vi "Laser Ops standalone diagnostics.vi"() -> ()   [LabVIEW 2017]
uses:
  Serial Comms/Visa resource.ctl
  Type Defs/Ls1 Operations.ctl
panel:
  out "Resp Validated (array) ?":bool[](array[boolean])
  out "Tmin":dbl
  out "Tmax":dbl
  out "Laser shutter":bool
  out "Ls Data":string[](array[string])
  out "error out inter":errorcluster
  out "error out":errorcluster
  in  "Program Stop":bool
  out "Pump peak hold":bool
  out "Power [mW]":dbl
  out "Read Wavelength [nm]":dbl
  in  "Laser Shutter":bool
  out "Tuning Status":string
  out "Fault":string
  out "Mode":string
  in  "PreChirper Available ?":bool
  in  "Laser Available ?":bool
  in  "Update":bool
  in  "Wavelength (nm)":u16
  in  "error in (no error)":errorcluster
  in  "PreChrp1 \nVisa resource":T1
  in  "Ls1 Visa \nresource":T1={"VISA resource name"="COM14", "baud rate"=19200}
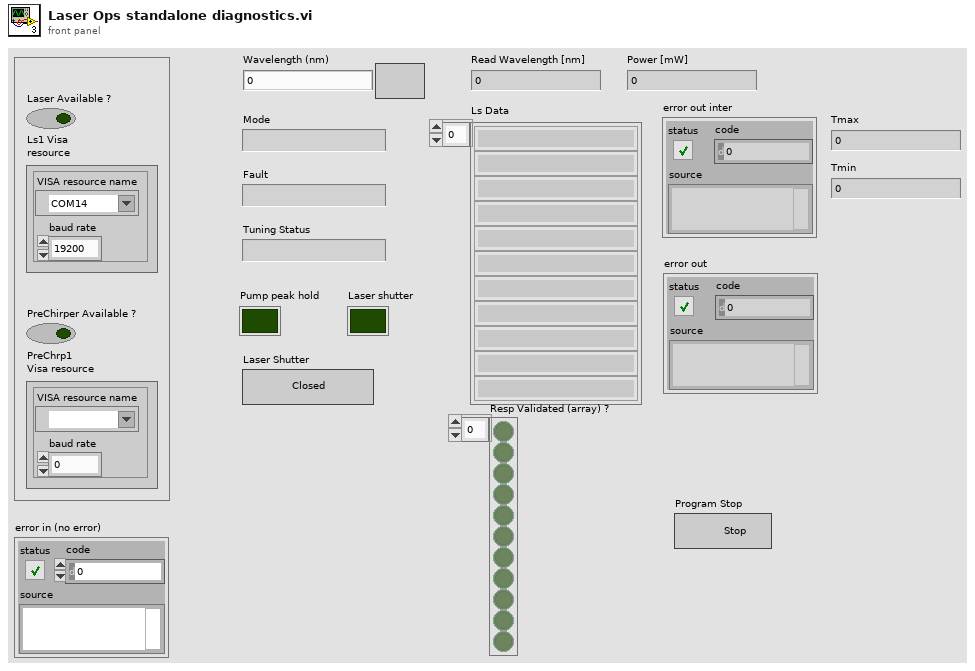
[diagram p1: front panel]
types:
  T1 = typedef "Visa resource.ctl" = cluster{"VISA resource name":refnum<visa-resource-name>, "baud rate":u32}
  T2 = typedef "Ls1 Operations.ctl" = enum16{"Initialise Connections", "Initialise system", "Check Status", "Open/Close Shutter", "Start/Stop Pump Peak Hold", "Set wavelength", "Close"}
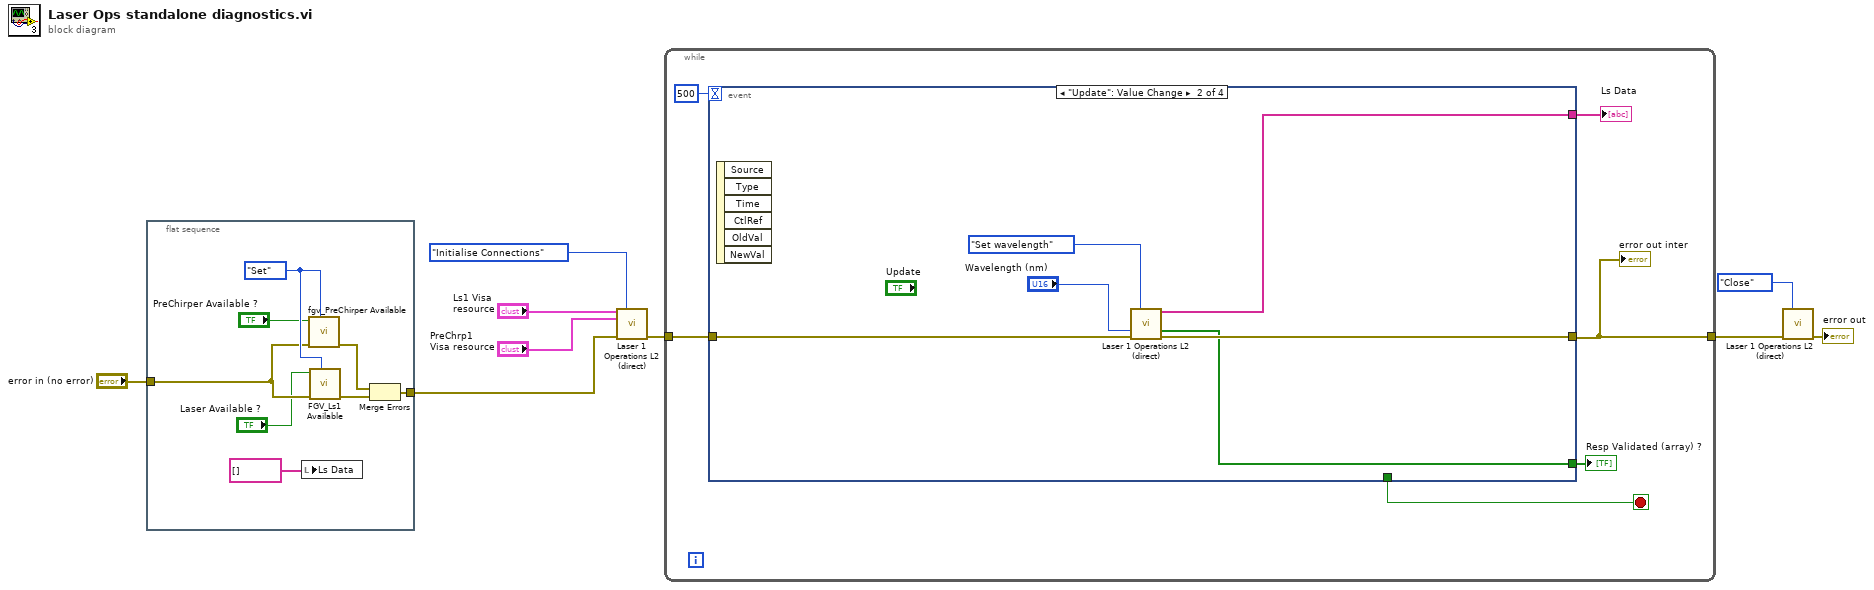
[diagram p0: block diagram]
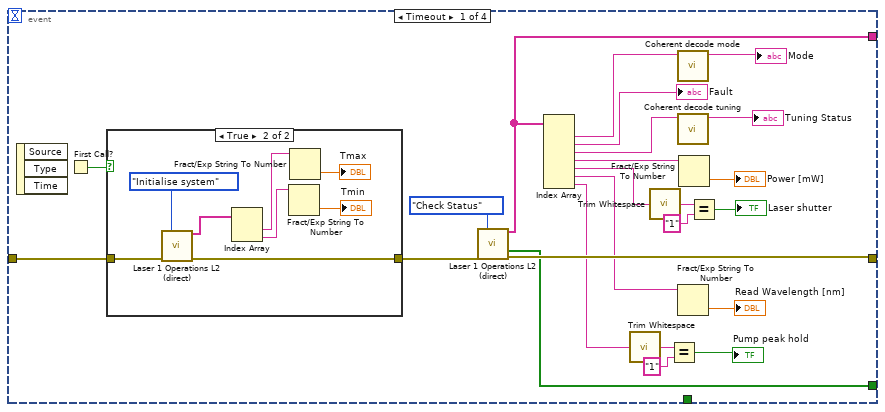
[diagram p2: hidden frame]
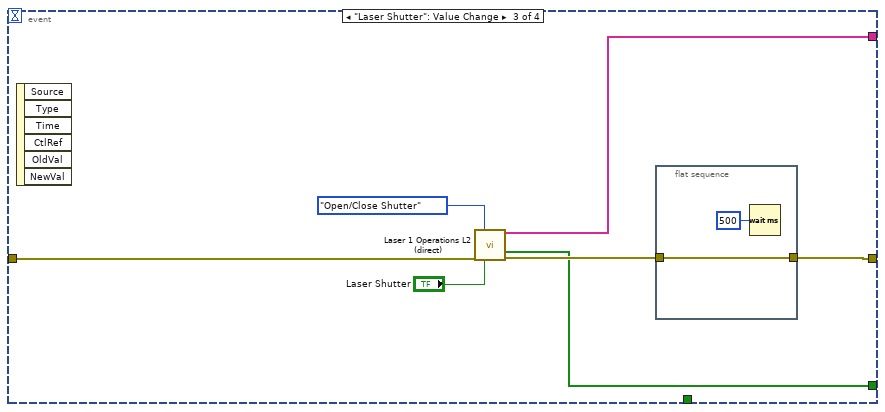
[diagram p4: hidden frame]
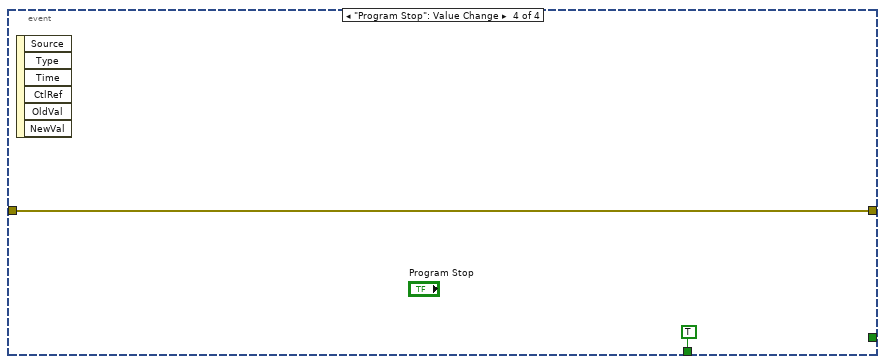
[diagram p5: hidden frame]
diagram:
  n1 = flat-sequence {
    tunnel: "error in (no error)" -> [w15]
    tunnel: [w12] -> w4
    frame #0 {
      w17 = enum16{"Get", "Set"}."Set" ("FGV Actions")
      n2 = local write "Ls Data"(string[] []) -> ()
      n3 = call "fgv_PreChirper Available.vi"("FGV Actions"=w17, "error in (no error)"=w15, "PreChirper Available ? IN"="PreChirper Available ?") -> ("error out"=w13:errorcluster)  [unwired: 7 in, 1 out]
      n4 = call "FGV_Ls1 Available.vi"("FGV Actions"=w17, "error in (no error)"=w15, "Laser Available ? IN"="Laser Available ?") -> ("error out"=w14:errorcluster)  [unwired: 7 in, 1 out]
      n5 = Merge Errors(w13, w14) -> (w12:errorcluster)
    }
  }
  n6 = call "Laser 1 Operations L2 (direct).vi"("Ls1 Visa \nresource"="Ls1 Visa \nresource", "Laser Ops\n actions"=Ls1_Operations."Initialise Connections" ("Laser Ops\n actions"), "PreChrp1 \nVisa resource"="PreChrp1 \nVisa resource", "error in (no error)"=w4) -> ("error out"=w6:errorcluster)  [unwired: 6 in, 5 out]
  n7 = while {
    tunnel: w6 -> [w23]
    tunnel: [w20] -> w2
    stop <- w21 stop-if-true
    n8 = event shown="[1] \"Update\": Value Change" {
      selector: _ -> [_ _ _ _]
      dyn-events: _ -> [_ _ _ _]
      timeout: 500 -> [_ _ _ _]
      tunnel: w23 -> [w46 w62 w68 w72]
      tunnel: [w44 w61 w64 w72] -> w20
      tunnel: [_ _ _ TRUE] -> w21
      tunnel: [w30 w58 w66 _] -> w19
      tunnel: [w24 w57 w63 _] -> w18
      event Timeout {
        n9 = event-data() -> ()  [unwired: 1 in, 3 out]
        n10 = First Call?() -> (First Call?: T/F=w47:bool)
        n11 = case shown="True" w47 {
          tunnel: w46 -> [w48 w56]
          tunnel: [w48 w49] -> w45
          frame False {
          }
          frame True {
            n12 = call "Laser 1 Operations L2 (direct).vi"("Laser Ops\n actions"=Ls1_Operations."Initialise system" ("Laser Ops\n actions"), "error in (no error)"=w56) -> ("Ls Data"=w54:string[], "error out"=w49:errorcluster)  [unwired: 8 in, 4 out]
            n13 = Index Array(array=w54) -> (element #1=w53:string, element #2=w52:string)  [unwired: 2 in]
            n14 = Fract/Exp String To Number(string=w52) -> (number=→"Tmin":dbl)  [unwired: 3 in, 1 out]
            n15 = Fract/Exp String To Number(string=w53) -> (number=→"Tmax":dbl)  [unwired: 3 in, 1 out]
          }
        }
        n16 = call "Laser 1 Operations L2 (direct).vi"("Laser Ops\n actions"=Ls1_Operations."Check Status" ("Laser Ops\n actions"), "error in (no error)"=w45) -> ("Ls Data"=w30:string[], "Resp Validated (array) ?"=w24:bool[], "error out"=w44:errorcluster)  [unwired: 8 in, 3 out]
        n17 = Index Array(array=w30) -> (element #1=w29:string, element #2=→"Fault":string, element #3=w27:string, element #4=w41:string, element #5=w37:string, element #6=w36:string, element #7=w32:string)  [unwired: 7 in]
        n18 = call <vilib>:"Trim Whitespace.vi"("string"=w32) -> ("trimmed string"=w34:string)  [unwired: 1 in]
        n19 = call <vilib>:"Trim Whitespace.vi"("string"=w37) -> ("trimmed string"=w39:string)  [unwired: 1 in]
        n20 = Equal?(x=w34, y="1") -> (x = y?=→"Pump peak hold":bool)
        n21 = call "Coherent decode mode.vi"("Mode string"=w29) -> ("Mode Desc."=→"Mode":string)  [unwired: 10 in]
        n22 = call "Coherent decode tuning.vi"("Tuning string"=w27) -> ("Tuning Desc."=→"Tuning Status":string)  [unwired: 10 in]
        n23 = Fract/Exp String To Number(string=w36) -> (number=→"Read Wavelength [nm]":dbl)  [unwired: 3 in, 1 out]
        n24 = Fract/Exp String To Number(string=w41) -> (number=→"Power [mW]":dbl)  [unwired: 3 in, 1 out]
        n25 = Equal?(x=w39, y="1") -> (x = y?=→"Laser shutter":bool)
      }
      event "Update": Value Change {
        n26 = event-data() -> ()  [unwired: 1 in, 6 out]
        n27 = call "Laser 1 Operations L2 (direct).vi"("Laser Ops\n actions"=Ls1_Operations."Set wavelength" ("Laser Ops\n actions"), "Wavelength \n(set) [nm]"="Wavelength (nm)", "error in (no error)"=w62) -> ("Ls Data"=w58:string[], "Resp Validated (array) ?"=w57:bool[], "error out"=w61:errorcluster)  [unwired: 7 in, 3 out]
      }
      event "Laser Shutter": Value Change {
        n28 = event-data() -> ()  [unwired: 1 in, 6 out]
        n29 = call "Laser 1 Operations L2 (direct).vi"("Laser Ops\n actions"=Ls1_Operations."Open/Close Shutter" ("Laser Ops\n actions"), "error in (no error)"=w68, "Boolean I/P"="Laser Shutter") -> ("Ls Data"=w66:string[], "Resp Validated (array) ?"=w63:bool[], "error out"=w65:errorcluster)  [unwired: 7 in, 3 out]
        n30 = flat-sequence {
          tunnel: w65 -> [w71]
          tunnel: [w71] -> w64
          frame #0 {
            n31 = Wait (ms)(milliseconds to wait=u32 500) -> ()  [unwired: 1 out]
          }
        }
      }
      event "Program Stop": Value Change {
        n32 = event-data() -> ()  [unwired: 1 in, 6 out]
      }
    }
    "error out inter" <- w20
    "Ls Data" <- w19
    "Resp Validated (array) ?" <- w18
  }
  n33 = call "Laser 1 Operations L2 (direct).vi"("Laser Ops\n actions"=Ls1_Operations."Close" ("Laser Ops\n actions"), "error in (no error)"=w2) -> ("error out"=→"error out":errorcluster)  [unwired: 8 in, 5 out]
